vi "DIOGenerator.vi"(1 "ValueIn":bool, 2 "Direction":bool, 3 "Index":u8) -> (0 "ValueOut":bool)   [LabVIEW 2019]
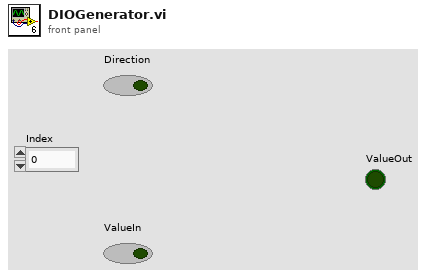
[diagram p1: front panel]
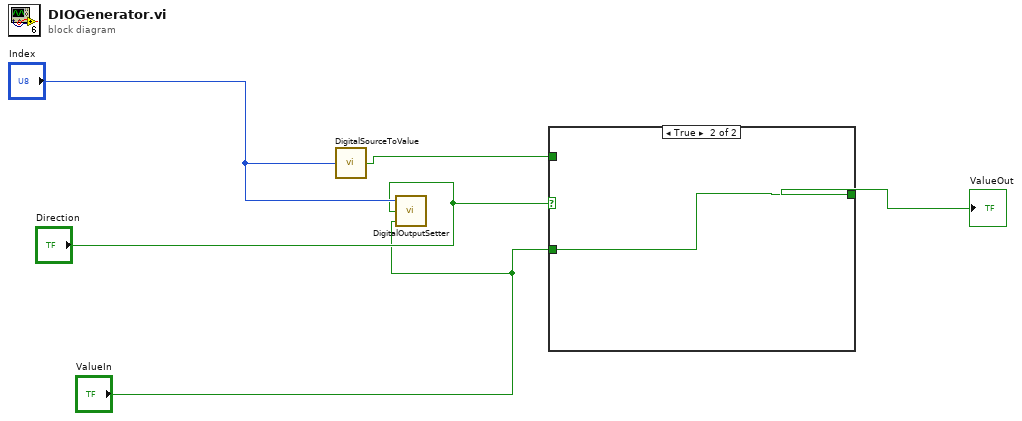
[diagram p0: block diagram]
diagram:
  n1 = call "DigitalSourceToValue.vi"("Index"="Index") -> ("Value"=w5:bool)
  n2 = call "DigitalOutputSetter.vi"("Value"="ValueIn", "Direction"="Direction", "Index"="Index") -> ()
  n3 = case shown="True" "Direction" {
    tunnel: "ValueIn" -> [_ w7]
    tunnel: w5 -> [w6 _]
    tunnel: [w6 w7] -> w4
    frame False {
    }
    frame True {
    }
  }
  "ValueOut" <- w4
